vi "Set Channel.vi"(8 "error in (no error)":errorcluster, 10 "Channel":T1, 11 "2936r in":refnum<class "2936r.lvclass">) -> (0 "error out":errorcluster, 3 "2936r out":refnum<class "2936r.lvclass">)   [LabVIEW 2018, in "2936r.lvlib" / "2936r.lvclass"]
uses:
  2936r.lvclass
  PPLs/Optical Power Meter/Optical Power Meter.lvlibp/Custom Controls/Channel List.ctl
  2936r.lvclass/2936r.ctl
  PPLs/Optical Power Meter/Optical Power Meter.lvlibp
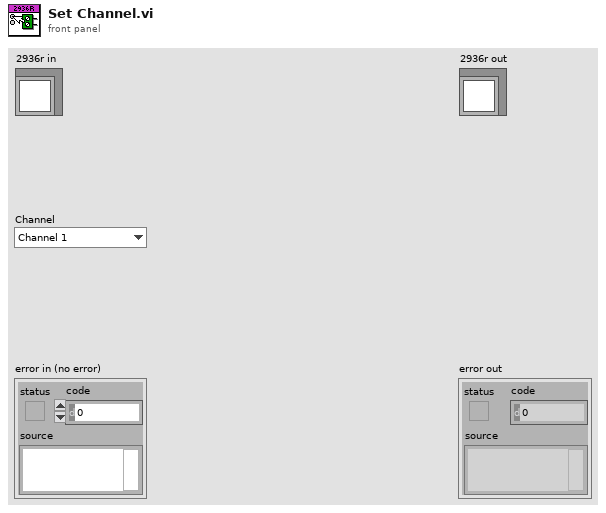
[diagram p1: front panel]
types:
  T1 = typedef "Optical Power Meter.lvlibp/Channel List.ctl" = enum16{"Channel 1", "Channel 2", "Channel 3", "Channel 4"}
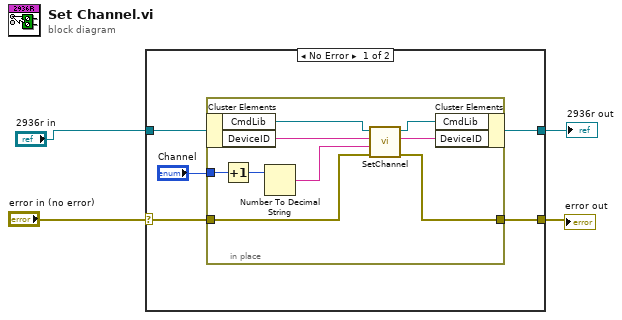
[diagram p0: block diagram]
diagram:
  n1 = case shown="No Error" "error in (no error)" {
    selector: "error in (no error)" -> [w7 w19]
    tunnel: "2936r in" -> [w9 w20]
    tunnel: [w6 w20] -> w2
    tunnel: [w5 w19] -> w1
    frame No Error {
      n2 = in-place {
        in-place-border: [w18] -> w5
        in-place-border: "Channel" -> [w17]
        in-place-border: w7 -> [w15]
        n3 = in-place-cluster #1(w9) -> ("CmdLib"=w13:refnum<k24>, "DeviceID"=w12:string)
        n4 = Increment(x=w17) -> (x+1=w16:T1)
        n5 = Number To Decimal String(number=w16) -> (decimal integer string=w14:string)  [unwired: 1 in]
        n6 = call <instrlib>:"SetChannel.vi"("error in"=w15, "Channel 1 or 2"=w14, "Device Key In"=w12, "PM Cmds In"=w13) -> ("error out"=w18:errorcluster, "Device Key Out"=w10:string, "PM Cmds Out"=w11:refnum<k24>)  [unwired: 1 in]
        n7 = in-place-cluster #1("CmdLib"=w11, "DeviceID"=w10) -> (w6:refnum<class "2936r.lvclass">)
      }
    }
    frame Error {
    }
  }
  "error out" <- w1
  "2936r out" <- w2
